vi "通信原理实验任务 1_4何德轩.vi"() -> ()   [LabVIEW 2018]
uses:
  <vilib>/measure/NI_MABase.lvlib
panel:
  in  "选项卡控件":enum32{"三个波形", "加噪声后的已调信号"}(tab)
  out "已调信号":waveform(dbl)(graph)
  out "载波":waveform(dbl)(graph)
  out "调制信号":waveform(dbl)(graph)
  out "加噪已调信号":waveform(dbl)[](graph)
  in  "载波":cluster{"载波频率(Hz)":dbl, "载波信号幅度(V)":dbl}={"载波频率(Hz)"=6000.0, "载波信号幅度(V)"=1.0}
  in  "调制信号":cluster{"调制频率(Hz)":dbl, "调制信号幅度(V)":dbl}={"调制频率(Hz)"=300.0, "调制信号幅度(V)"=10.0}
  in  "噪声":cluster{"噪声幅度(V)":dbl}={"噪声幅度(V)"=2.0}
  in  "采样参数":cluster{"采样率(Hz)":dbl, "采样数":dbl}={"采样率(Hz)"=300000.0, "采样数"=600000.0}
  # "参数设置面板"
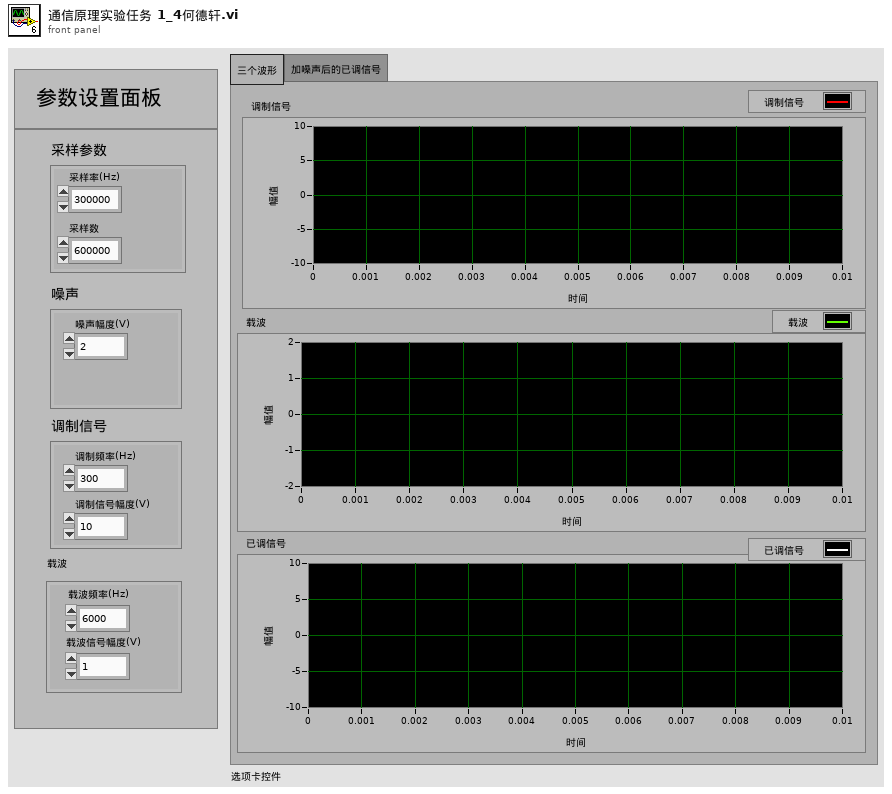
[diagram p1: front panel]
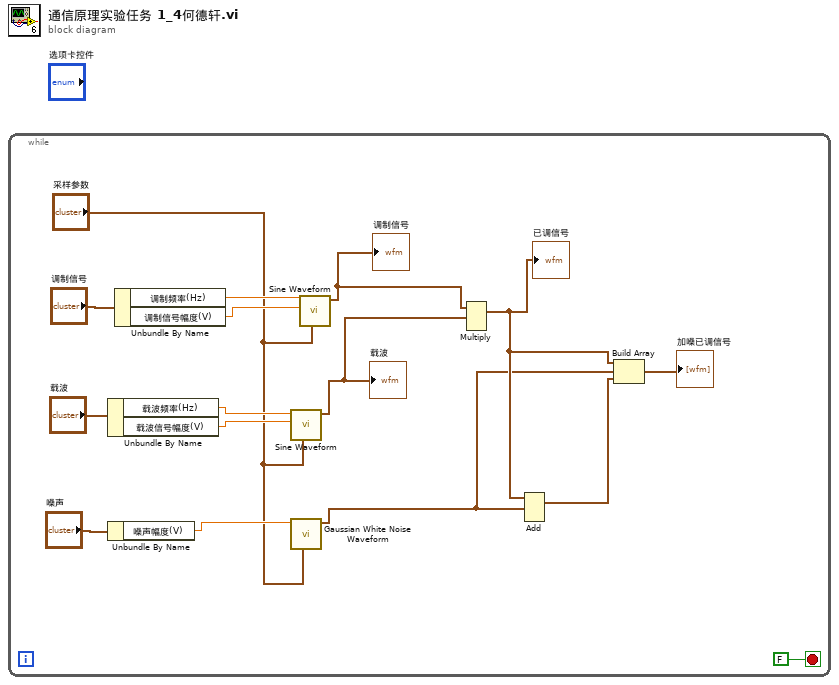
[diagram p0: block diagram]
diagram:
  n1 = while {
    stop <- FALSE stop-if-true
    n2 = Unbundle By Name("载波") -> ("载波频率(Hz)"=w11:dbl, "载波信号幅度(V)"=w10:dbl)
    n3 = Unbundle By Name("噪声") -> ("噪声幅度(V)"=w9:dbl)
    n4 = Unbundle By Name("调制信号") -> ("调制频率(Hz)"=w13:dbl, "调制信号幅度(V)"=w12:dbl)
    n5 = call <vilib>:"Sine Waveform.vi"("sampling info"="采样参数", "amplitude"=w10, "frequency"=w11) -> ("signal out"=w6:waveform(dbl))  [unwired: 7 in, 1 out]
    "载波" <- w6
    n6 = call <vilib>:"Gaussian White Noise Waveform.vi"("sampling info"="采样参数", "standard deviation"=w9) -> ("signal out"=w4:waveform(dbl))  [unwired: 8 in, 1 out]
    n7 = call <vilib>:"Sine Waveform.vi"("sampling info"="采样参数", "amplitude"=w12, "frequency"=w13) -> ("signal out"=w7:waveform(dbl))  [unwired: 7 in, 1 out]
    "调制信号" <- w7
    n8 = Multiply(1:w6, 2:w7) -> (0:w5:waveform(dbl))  [unwired: 1 in, 1 out]
    "已调信号" <- w5
    n9 = Add(1:w4, 2:w5) -> (0:w3:waveform(dbl))  [unwired: 1 in, 1 out]
    n10 = Build Array(w5, w4, w3) -> (→"加噪已调信号":waveform(dbl)[])
  }
